vi "CameraQueryAcquire.vi"(8 "error in (no error)":errorcluster, 11 "NIvision in":refnum<class "IMAQdx_Flea3_Firewire.lvclass">) -> (0 "error out":errorcluster, 1 "frames_done":u32, 2 "acquiring":bool, 3 "NIvision out":refnum<class "IMAQdx_Flea3_Firewire.lvclass">)   [LabVIEW 2012, in "IMAQdx_Flea3_Firewire.lvclass"]
uses:
  <userlib>/BIAS2/classes/IMAQdx_Flea3_Firewire/IMAQdx_Flea3_Firewire.lvclass
  <userlib>/BIAS2/classes/IMAQdx_Flea3_Firewire/IMAQdx_Flea3_Firewire.lvclass/IMAQdx_Flea3_Firewire.ctl
  <resource>/objmgr/imaqdx.rc
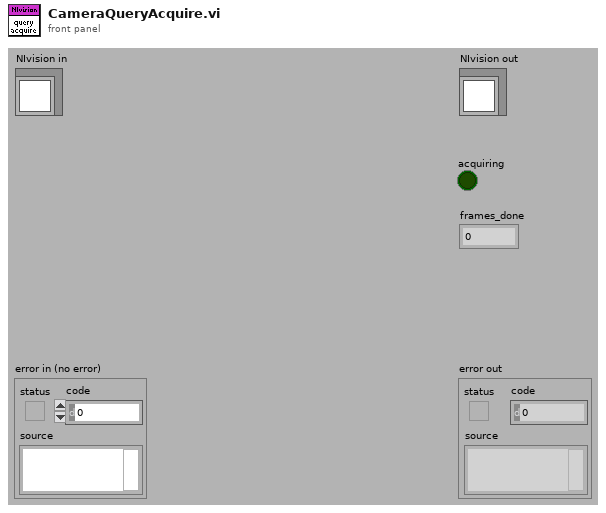
[diagram p1: front panel]
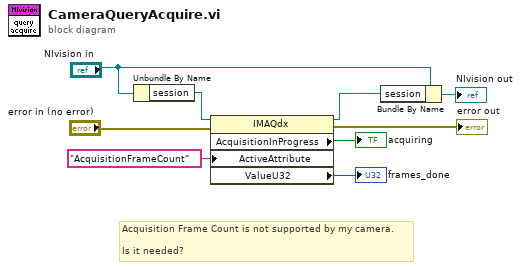
[diagram p0: block diagram]
diagram:
  # "Acquisition Frame Count is not supported by my camera.\n\nIs it needed?"
  n1 = Unbundle By Name("NIvision in") -> ("session"=w7:refnum<k21>)
  n2 = property class="IMAQdx"(reference=w7, error in="error in (no error)", "ActiveAttribute"="AcquisitionFrameCount") -> (reference out=w8:refnum<k21>, error out=→"error out":errorcluster, "AcquisitionInProgress"=→"acquiring":bool, "ValueU32"=→"frames_done":u32)
  n3 = Bundle By Name(cluster="NIvision in", "session"=w8) -> (→"NIvision out":refnum<class "IMAQdx_Flea3_Firewire.lvclass">)
